vi "Control Editor Panel.vi"(8 "error in (no error)":errorcluster, 10 "Control Type":string, 11 "Control List in":refnum<class "Control List.lvclass">) -> (0 "error out":errorcluster, 2 "Panel":refnum<class "ElementEditorPanel.lvclass">, 3 "Control List out":refnum<class "Control List.lvclass">)   [LabVIEW 2020, in "VolatusGUIEditor.lvlib" / "Control List.lvclass"]
uses:
  Control List.lvclass
  VolatusGUIEditorCore/ElementEditorPanel/ElementEditorPanel.lvclass
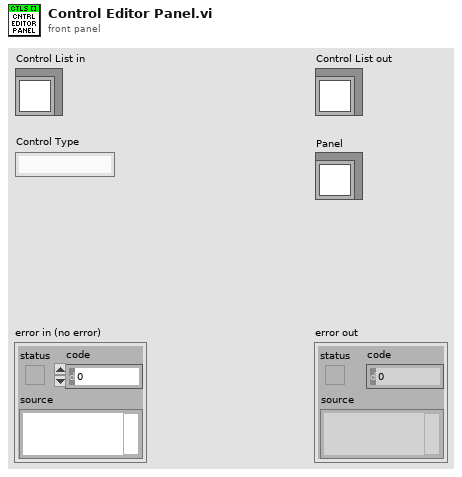
[diagram p1: front panel]
types:
  T1 = map{string, refnum<class "ElementEditorPanel.lvclass">}
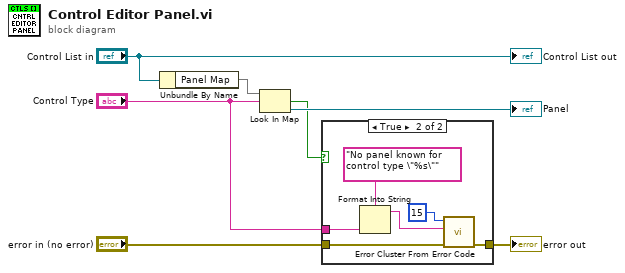
[diagram p0: block diagram]
diagram:
  n1 = Unbundle By Name("Control List in") -> ("Panel Map"=w6:T1)
  n2 = Look In Map(map=w6, key="Control Type") -> (key not found?=w4:bool, value=→"Panel":refnum<class "ElementEditorPanel.lvclass">)  [unwired: 1 in]
  n3 = case shown="True" w4 {
    tunnel: "error in (no error)" -> [w8 w12]
    tunnel: [w8 w11] -> w2
    tunnel: "Control Type" -> [_ w14]
    frame False {
    }
    frame True {
      n4 = Format Into String(format string="No panel known for control type \"%s\"", w14) -> (resulting string=w9:string)  [unwired: 2 in, 1 out]
      n5 = call <vilib>:"Error Cluster From Error Code.vi"("error in (no error)"=w12, "error message (\"\")"=w9, "error code (0)"=15) -> ("error out"=w11:errorcluster)  [unwired: 6 in]
    }
  }
  "error out" <- w2
  "Control List out" <- "Control List in"
